vi "Execution_StartProcess.vi"(8 "error in (no error)":errorcluster, 10 "Process in":refnum<class "Process.lvclass">, 11 "EVE reference in":refnum<data-value>) -> (0 "error out":errorcluster, 3 "EVE reference out":refnum<data-value>)   [LabVIEW 2013, in "Process.lvclass"]
uses:
  Process.lvclass
  001 - MAIN/Class/EVE/EVE.lvclass
  090 - ERRORS/Ctrls/EnumErrors.ctl
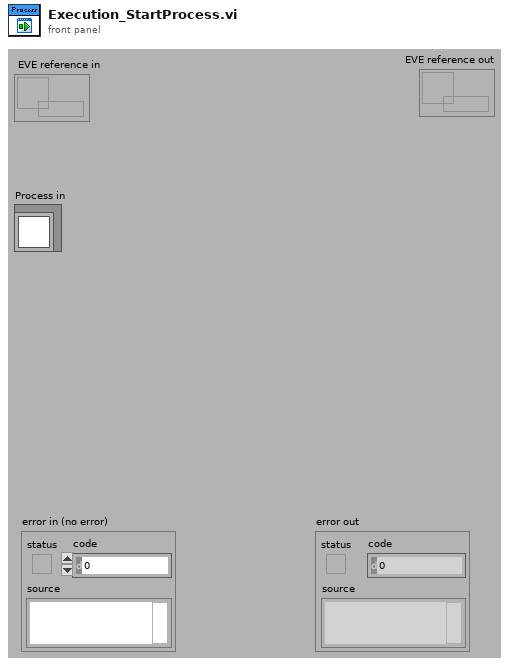
[diagram p1: front panel]
types:
  T1 = typedef "EnumErrors.ctl" = enum16{"VI non trouvé !", "Clé non trouvée", "Timeout", "Le VI tourne déjà", "Erreur de séparateur décimal", "Référence non trouvée"}
  T2 = typedef "FromProcessesEventType.ctl" = enum16{"Started", "Autotest", "Ended"}
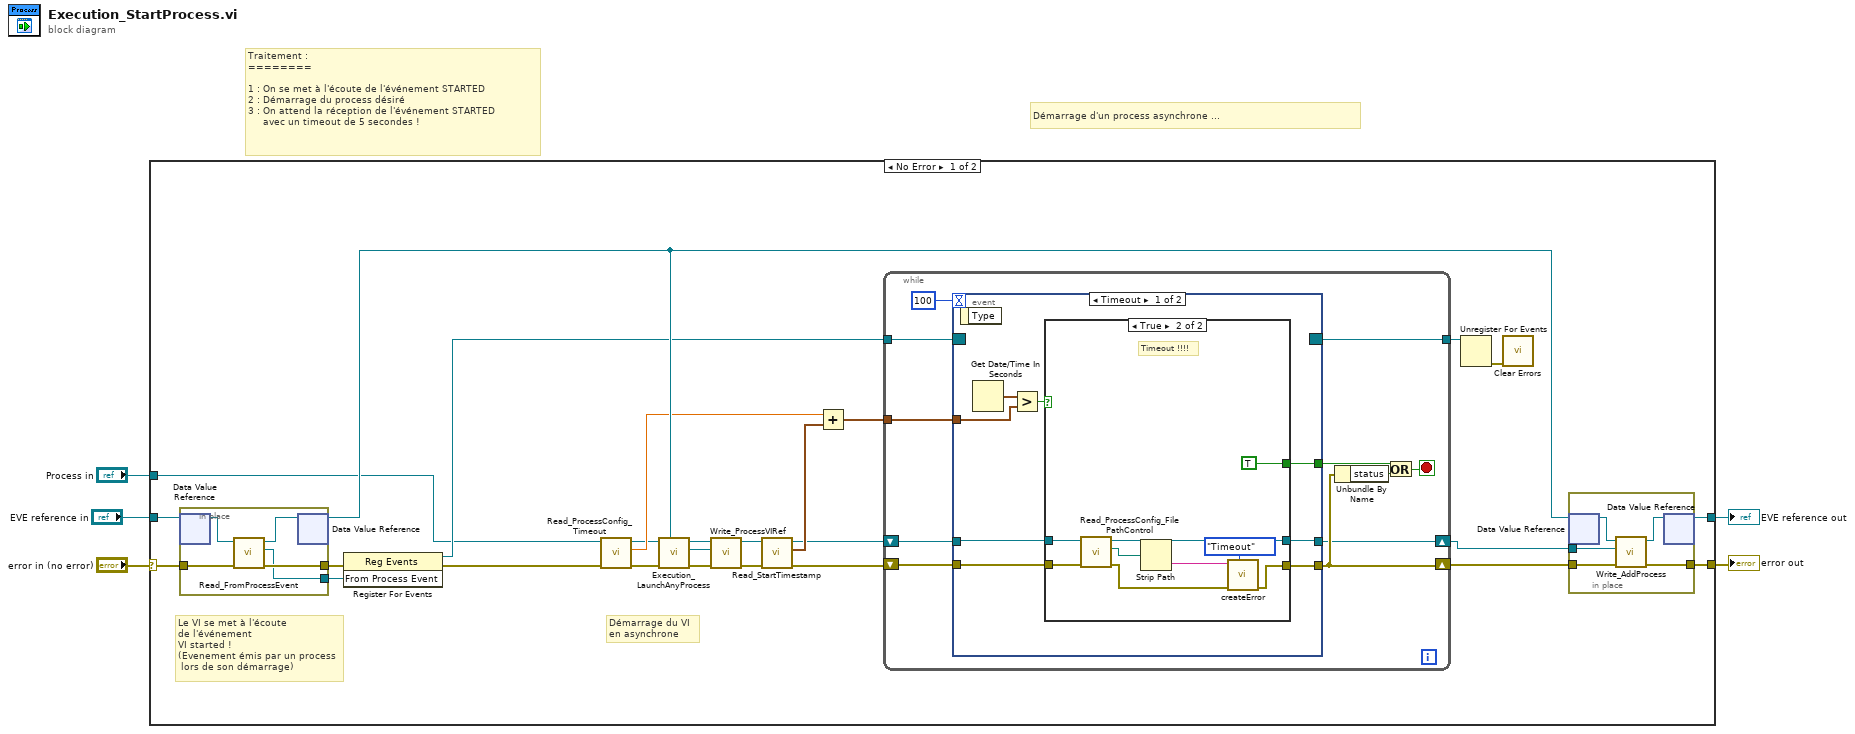
[diagram p0: block diagram]
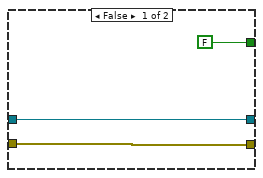
[diagram p2: hidden frame]
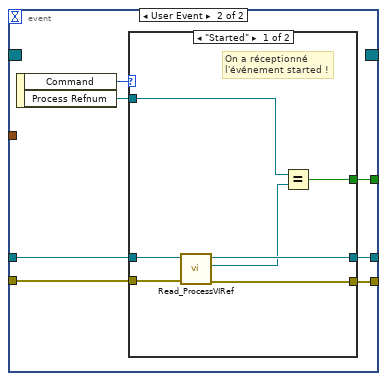
[diagram p3: hidden frame]
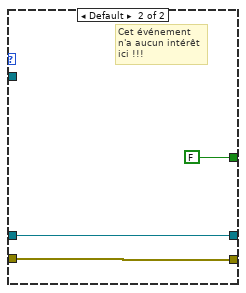
[diagram p4: hidden frame]
diagram:
  # "Traitement :\n========\n\n1 : On se met à l'écoute de l'événement STARTED\n2 : Démarrage du process désiré\n3 : On attend la réception de l'événement STARTED\n     avec un timeout de 5 secondes !"
  # "Démarrage d'un process asynchrone ..."
  n1 = case shown="No Error" "error in (no error)" {
    selector: "error in (no error)" -> [w21 w91]
    tunnel: [w22 w91] -> w5
    tunnel: "EVE reference in" -> [w9 w90]
    tunnel: [w8 w90] -> w1
    tunnel: "Process in" -> [w6 _]
    frame No Error {
      # "Le VI se met à l'écoute\nde l'événement \nVI started !\n(Evenement émis par un process\n lors de son démarrage)"
      # "Démarrage du VI \nen asynchrone"
      n2 = in-place {
        in-place-border: [w41] -> w29
        in-place-border: [w40] -> w24
        in-place-border: w21 -> [w39]
        n3 = in-place-dvr #1(w9) -> (w38:refnum<class "EVE.lvclass">)  [unwired: 1 out]
        n4 = call "Read_FromProcessEvent.vi"("error in (no error)"=w39, "EVE.lvclass in"=w38) -> ("error out"=w41:errorcluster, "From Process Event"=w40:refnum<user-event>, "EVE.lvclass out"=w37:refnum<class "EVE.lvclass">)  [unwired: 7 in]
        n5 = in-place-dvr #1(w37) -> (w31:refnum<data-value>)  [unwired: 1 out]
      }
      n6 = register-events(error in=w29, w24) -> (reference out=w25:refnum<event-registration>, error out=w7:errorcluster)  [unwired: 1 in]
      n7 = call-dynamic "Read_ProcessConfig_Timeout.vi"("error in (no error)"=w7, "Process in"=w6) -> ("error out"=w16:errorcluster, "Timeout"=w15:dbl, "Process out"=w12:refnum<class "Process.lvclass">)  [unwired: 7 in]
      n8 = call-dynamic "Execution_LaunchAnyProcess.vi"("EVE reference in"=w31, "error in (no error)"=w16, "Process in"=w12) -> ("error out"=w20:errorcluster, "vi reference"=w18:refnum<vi>, "Process out"=w19:refnum<class "Process.lvclass">)  [unwired: 6 in]
      n9 = call-dynamic "Write_ProcessVIRef.vi"("error in (no error)"=w20, "Process VI Ref"=w18, "Process in"=w19) -> ("error out"=w13:errorcluster, "Process out"=w14:refnum<class "Process.lvclass">)  [unwired: 7 in]
      n10 = call-dynamic "Read_StartTimestamp.vi"("error in (no error)"=w13, "Process in"=w14) -> ("error out"=w11:errorcluster, "Start Timestamp"=w30:timestamp, "Process out"=w10:refnum<class "Process.lvclass">)  [unwired: 7 in]
      n11 = Add(x=w15, y=w30) -> (x+y=w28:timestamp)
      n12 = while {
        tunnel: w25 -> [w52]
        shift-right: [w48] -> w23
        shift-left: w11 -> [w44]
        tunnel: w28 -> [w51]
        tunnel: [w50] -> w27
        shift-right: [w42] -> w17
        shift-left: w10 -> [w43]
        stop <- w45 stop-if-true
        n13 = event shown="[0] Timeout" {
          selector: w52 -> [_ _]
          dyn-events: [_ _] -> w50
          timeout: 100 -> [_ _]
          tunnel: w44 -> [w58 w77]
          tunnel: [w56 w76] -> w48
          tunnel: w51 -> [w59 _]
          tunnel: [w55 w78] -> w46
          tunnel: w43 -> [w54 w73]
          tunnel: [w53 w74] -> w42
          event Timeout {
            n14 = event-data() -> ()  [unwired: 1 in, 1 out]
            n15 = Get Date/Time In Seconds() -> (seconds since 1Jan1904=w60:timestamp)
            n16 = Greater?(x=w60, y=w59) -> (0:w57:bool)
            n17 = case shown="True" w57 {
              tunnel: w58 -> [w63 w68]
              tunnel: [w63 w71] -> w56
              tunnel: [FALSE TRUE] -> w55
              tunnel: w54 -> [w61 w65]
              tunnel: [w61 w64] -> w53
              frame False {
              }
              frame True {
                # "Timeout !!!!"
                n18 = call-dynamic "Read_ProcessConfig_File PathControl.vi"("error in (no error)"=w68, "Process in"=w65) -> ("error out"=w67:errorcluster, "File Path Control"=w66:path, "Process out"=w64:refnum<class "Process.lvclass">)  [unwired: 7 in]
                n19 = Strip Path(path=w66) -> (name=w69:string)  [unwired: 1 out]
                n20 = call "createError.vi"("ErrorCode"=EnumErrors."Timeout", "error in"=w67, "message"=w69) -> ("error out"=w71:errorcluster)  [unwired: 8 in]
              }
            }
          }
          event User Event {
            n21 = event-data() -> ("Command"=w79:T2, "Process Refnum"=w75:refnum<vi>)  [unwired: 1 in]
            n22 = case shown="\"Started\"" w79 {
              tunnel: [w85 FALSE] -> w78
              tunnel: w77 -> [w82 w88]
              tunnel: [w81 w88] -> w76
              tunnel: w75 -> [w86 _]
              tunnel: [w83 w87] -> w74
              tunnel: w73 -> [w84 w87]
              frame "Started" {
                # "On a réceptionné \nl'événement started !"
                n23 = call-dynamic "Read_ProcessVIRef.vi"("error in (no error)"=w82, "Process in"=w84) -> ("error out"=w81:errorcluster, "Process VI Ref"=w80:refnum<vi>, "Process out"=w83:refnum<class "Process.lvclass">)  [unwired: 7 in]
                n24 = Equal?(x=w86, y=w80) -> (x = y?=w85:bool)
              }
              frame Default {
                # "Cet événement \nn'a aucun intérêt\nici !!!"
              }
            }
          }
        }
        n25 = Unbundle By Name(w48) -> ("status"=w47:bool)
        n26 = Or(x=w46, y=w47) -> (x .or. y?=w45:bool)
      }
      n27 = Unregister For Events(event registration refnum=w27) -> (error out=w26:errorcluster)  [unwired: 1 in]
      n28 = call <vilib>:"Clear Errors.vi"("error in (no error)"=w26) -> ()  [unwired: 6 in, 1 out]
      n29 = in-place {
        in-place-border: w23 -> [w36]
        in-place-border: [w35] -> w22
        in-place-border: w17 -> [w34]
        n30 = in-place-dvr #2(w31) -> (w33:refnum<class "EVE.lvclass">)  [unwired: 1 out]
        n31 = call "Write_AddProcess.vi"("error in (no error)"=w36, "Process in"=w34, "EVE.lvclass in"=w33) -> ("error out"=w35:errorcluster, "EVE.lvclass out"=w32:refnum<class "EVE.lvclass">)  [unwired: 7 in]
        n32 = in-place-dvr #2(w32) -> (w8:refnum<data-value>)  [unwired: 1 out]
      }
    }
    frame Error {
    }
  }
  "error out" <- w5
  "EVE reference out" <- w1
